vi "DAQ Configuration to JSON.vi"(8 "error in":errorcluster, 11 "DAQmx Configuration":T1={"Run Mode"=0, "Sample Rate (Hz)"=51200.0, "Block Size"=5120, "Channel Table"=[], "Trigger Type"=0, "Trigger Channel"="", "Level"=1.0, "Pretrigger"=20, "Hysteresis"=0.0, "Slope"=enum."Rising"} {"Run Mode" items=["Run Once", "Continuously"]; "Block Size" min=0; "Sample Rate (Hz)" min=0.0; "Trigger Type" items=["None", "Analog Reference"]; "Channel Table"."input terminal configuration" items=["default"=-1, "RSE"=10083, "NRSE"=10078, "Differential"=10106, "Pseudodifferential"=12529]; "Channel Table"."Channel Type" items=["Voltage (V)"=0, "Charge (C)"=9, "-"=99, "SPL (Pa)"=3, "Force (lbf)"=6, "Force (N)"=1, "Acceleration (g) - IEPE"=2, "Acceleration (g) - Charge"=12, "Acceleration (g) - 4 wire DC Voltage"=22, "Velocity (in/s)"=7, "Velocity (mm/s)"=8, "Prox Probe (mil)"=4, "Prox Probe (mm)"=5]}) -> (0 "error out":errorcluster, 3 "flattened JSON configuration":string)   [LabVIEW 2024, in "Dynamic Signal Acquisition (Interactive) UI.lvlib"]
uses:
  Dynamic Signal Acquisition (Interactive) UI.lvlib
  SFPDAQ Configuration.ctl
  SFPDAQmx Channel Info.ctl
  <vilib>/JDP Science/JSONtext/JSONtext.lvlib
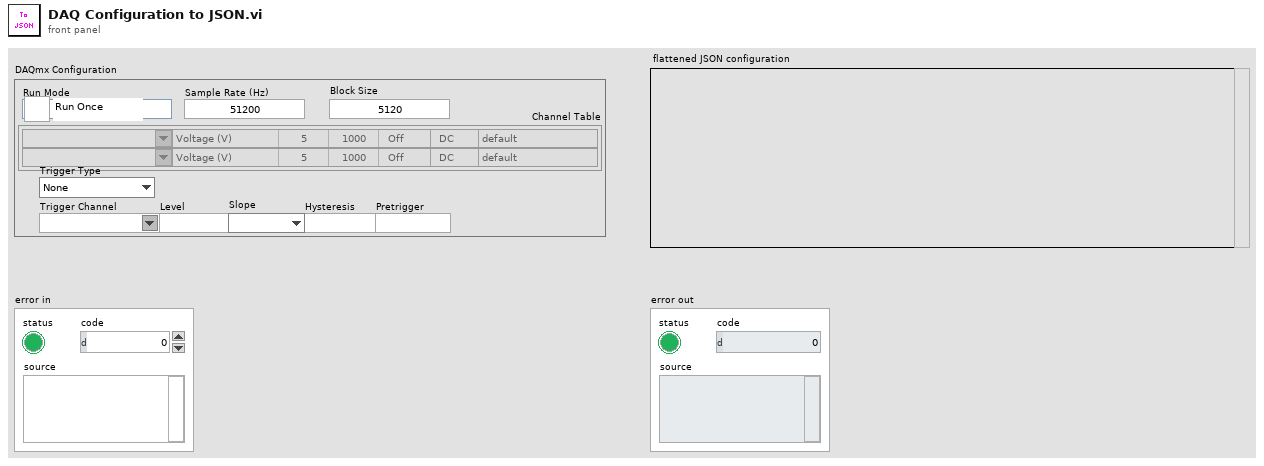
[diagram p1: front panel]
types:
  T1 = typedef "Dynamic Signal Acquisition (Interactive) UI.lvlib/SFPDAQ Configuration.ctl" = cluster{"Run Mode":u16, "Sample Rate (Hz)":dbl, "Block Size":i32, "Channel Table":T2[], "Trigger Type":u16, "Trigger Channel":string, "Level":dbl, "Pretrigger":i32, "Hysteresis":dbl, "Slope":enum16{"Falling", "Rising"}}
  T2 = typedef "Dynamic Signal Acquisition (Interactive) UI.lvlib/SFPDAQmx Channel Info.ctl" = cluster{"DAQmx Channel":tag, "Channel Type":u16, "Max":dbl, "Sensitivity":dbl, "Coupling":enum16{"AC", "DC"}, "input terminal configuration":i32, "excitation":enum16{"Off", "Min", "Max"}}
  T3 = cluster{"Run Mode":u16, "Sample Rate (Hz)":dbl, "Block Size":i32, "Channel Table":cluster{"DAQmx Channel":string, "Channel Type":u16, "Max":dbl, "Sensitivity":dbl, "Coupling":string, "input terminal configuration":i32, "excitation value":string}[], "Trigger Type":u16, "Trigger Channel":string, "Level":dbl, "Pretrigger":i32, "Hysteresis":dbl, "Slope":string}
  T4 = cluster{"DAQmx Channel":string, "Channel Type":u16, "Max":dbl, "Sensitivity":dbl, "Coupling":string, "input terminal configuration":i32, "excitation value":string}
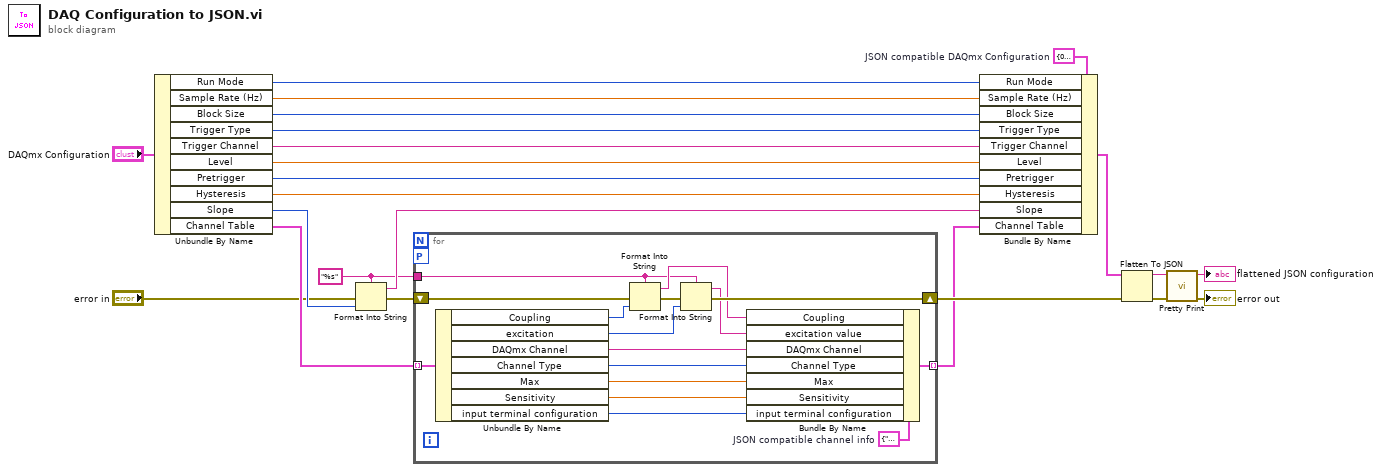
[diagram p0: block diagram]
diagram:
  w8 = "%s" ("format string")
  w19 = T3 {"Run Mode"=0, "Sample Rate (Hz)"=51200.0, "Block Size"=5120, "Channel Table"=[], "Trigger Type"=0, "Trigger Channel"="", "Level"=0.0, "Pretrigger"=20, "Hysteresis"=0.0, "Slope"=""}  # JSON compatible DAQmx Configuration
  n1 = Unbundle By Name("DAQmx Configuration") -> ("Run Mode"=w1:u16, "Sample Rate (Hz)"=w15:dbl, "Block Size"=w14:i32, "Trigger Type"=w13:u16, "Trigger Channel"=w12:string, "Level"=w11:dbl, "Pretrigger"=w10:i32, "Hysteresis"=w9:dbl, "Slope"=w20:enum16{"Falling", "Rising"}, "Channel Table"=w22:T2[])
  n2 = Format Into String(format string=w8, error in="error in", w20) -> (resulting string=w18:string, error out=w6:errorcluster)  [unwired: 1 in]
  n3 = for {
    tunnel: w22 -> [w34] mode=indexing
    workers-P: _ -> [_]
    shift-right: [w37] -> w21
    shift-left: w6 -> [w39]
    tunnel: [w30] -> w17 mode=indexing
    tunnel: w8 -> [w24]
    w33 = T4 {"DAQmx Channel"="", "Channel Type"=0, "Max"=5.0, "Sensitivity"=1000.0, "Coupling"="", "input terminal configuration"=-1, "excitation value"=""}  # JSON compatible channel info
    n4 = Unbundle By Name(w34) -> ("Coupling"=w36:enum16{"AC", "DC"}, "excitation"=w35:enum16{"Off", "Min", "Max"}, "DAQmx Channel"=w29:tag, "Channel Type"=w28:u16, "Max"=w27:dbl, "Sensitivity"=w26:dbl, "input terminal configuration"=w25:i32)
    n5 = Format Into String(format string=w24, error in=w39, w36) -> (resulting string=w32:string, error out=w38:errorcluster)  [unwired: 1 in]
    n6 = Format Into String(format string=w24, error in=w38, w35) -> (resulting string=w31:string, error out=w37:errorcluster)  [unwired: 1 in]
    n7 = Bundle By Name(cluster=w33, "Coupling"=w32, "excitation value"=w31, "DAQmx Channel"=w29, "Channel Type"=w28, "Max"=w27, "Sensitivity"=w26, "input terminal configuration"=w25) -> (w30:T4)
  }
  n8 = Bundle By Name(cluster=w19, "Run Mode"=w1, "Sample Rate (Hz)"=w15, "Block Size"=w14, "Trigger Type"=w13, "Trigger Channel"=w12, "Level"=w11, "Pretrigger"=w10, "Hysteresis"=w9, "Slope"=w18, "Channel Table"=w17) -> (w16:T3)
  n9 = Flatten To JSON(anything=w16, error in (no error)=w21) -> (JSON string=w5:string, 11:w3:errorcluster)  [unwired: 1 in]
  n10 = call <vilib>:"Pretty Print.vi"("error in (no error)"=w3, "JSON"=w5) -> ("error out"=→"error out":errorcluster, "<JSON>"=→"flattened JSON configuration":string)  [unwired: 7 in, 1 out]
